vi "SDT_WriteFileDecayFCSMCS.vi"(5 "ActiveModule":string[](array[string]), 7 "FCSFileData":T1, 8 "ErrorIn":errorcluster, 9 "SPCdata":T14={"base_adr"=0, "init"=0, "cfd_limit_low"=0.0, "cfd_limit_high"=0.0, "cfd_zc_level"=0.0, "cfd_holdoff"=0.0, "sync_zc_level"=0.0, "sync_holdoff"=0.0, "sync_threshold"=0.0, "tac_range"=0.0, "sync_freq_div"=0, "tac_gain"=0, "tac_offset"=0.0, "tac_limit_low"=0.0, "tac_limit_high"=0.0, "adc_resolution"=12, "ext_latch_delay"=0, "collect_time"=0.0, "display_time"=0.0, "repeat_time"=0.0, "stop_on_time"=0, "stop_on_ovfl"=0, "dither_range"=0, "count_incr"=0, "mem_bank"=0, "dead_time_comp"=0, "scan_control"=0, "routing_mode"=0, "tac_enable_hold"=0.0, "pci_card_no"=0, "mode"=0, "scan_size_x"=0, "scan_size_y"=0, "scan_rout_x"=0, "scan_rout_y"=0, "scan_flyback"=0, "scan_borders"=0, "scan_polarity"=0, "pixel_clock"=0, "line_compression"=0, "trigger"=0, "pixel_time"=0.0, "ext_pixclk_div"=0, "rate_count_time"=0.0, "macro_time_clk"=0, "add_select"=0, "test_eep"=0, "adc_zoom"=0, "img_size_x"=0, "img_size_y"=0, "img_rout_x"=0, "img_rout_y"=0, "xy_gain"=0, "master_clock"=0, "adc_sample_delay"=0, "detector_type"=0, "chan_enable"=0, "chan_slope"=0, "chan_spec_no"=0, "tdc_control"=0, "tdc_offset1"=0.0, "tdc_offset2"=0.0, "tdc_offset3"=0.0, "tdc_offset4"=0.0, "tdc_offset5"=0.0, "tdc_offset6"=0.0, "cfd_th5_tdc"=0.0, "cfd_th6_tdc"=0.0, "cfd_zc5_tdc"=0.0, "cfd_zc6_tdc"=0.0, "future_reserve1"=0, "future_reserve2"=0, "future_reserve3"=0, "future_reserve4"=0}, 10 "FileType":T2=2 items=["non-Fifo"=1, "Fifo"=2, "FifoImage"=3], 11 "SDT-FilePath":path=path "\\\\lab13\\C/Users/jannis/Desktop/ZeissFifo.sdt") -> (0 "ErrorOut":errorcluster)   [LabVIEW 2017]
doc: "This VI writes a SDT-file to disc. The SetUp and the MeasureInfo blocks are created and appended with the data blocks. \nThis VI is limited to writing a DecayMatrix from a FIFO-Image recording and optional an IntensityImage to file. For single mode recordings use the spcmdll VI \\Public\\Configure\\Memory Transfer\\SPC_save_data_to_sdtfile.vi.\nFor a description of the format for the Data input cluster to this VI see the usage in \\Example\\ImagingEventStream-SimpleFifoImage.vi. Leave either of the cluster input arrays empty to not save them to disc.\nFor a description of the *.sdt file format see: SPC_data_file_structure.h\n\ninfo@becker-hickl.com"
uses:
  SPC_Wrappers/SPC_Controls/bhfile_header.ctl
  SPC_Wrappers/SPC_Controls/SPCdata.ctl
  SPC_Wrappers/SPC_Controls/MeasureInfo.ctl
  SPC_Wrappers/SPC_Controls/MeasureInfo_PartB.ctl
  SPC_Wrappers/SPC_Controls/MeasStopInfo.ctl
  SPC_Wrappers/SPC_Controls/MeasFCSInfo.ctl
  SPC_Wrappers/SPC_Controls/MeasureInfo_PartE.ctl
  SPC_Wrappers/SPC_Controls/MeasHISTInfo.ctl
  SPC_Wrappers/SPC_Controls/HISTInfoExt.ctl
  SPC_Wrappers/SPC_Controls/MeasureInfo_PartI.ctl
  SPC_Wrappers/SPC_Controls/MeasureInfo_PartK.ctl
  SPC_Wrappers/SPC_Controls/MeasureInfo_PartM.ctl
  SPC_Wrappers/SPC_Controls/BHFileBlockHeader.ctl
  SPC_Wrappers/SPC_Controls/FileType.ctl
  SDT_CreateModTypeString.vi
  SDT_MeasureBlockToString.vi
panel:
  out "Info Block":string
  out "BHFileBlockHeaders":T3[](array[typedef])
  out "MeasureInfos":T4 {"MeasStopInfo"."flags" format="x%x"}
  out "ArrayLengths":i32[](array[numeric])
  out "bhfile_header":T15 {"chksum" format="x%x"; "header_valid" format="x%x"}
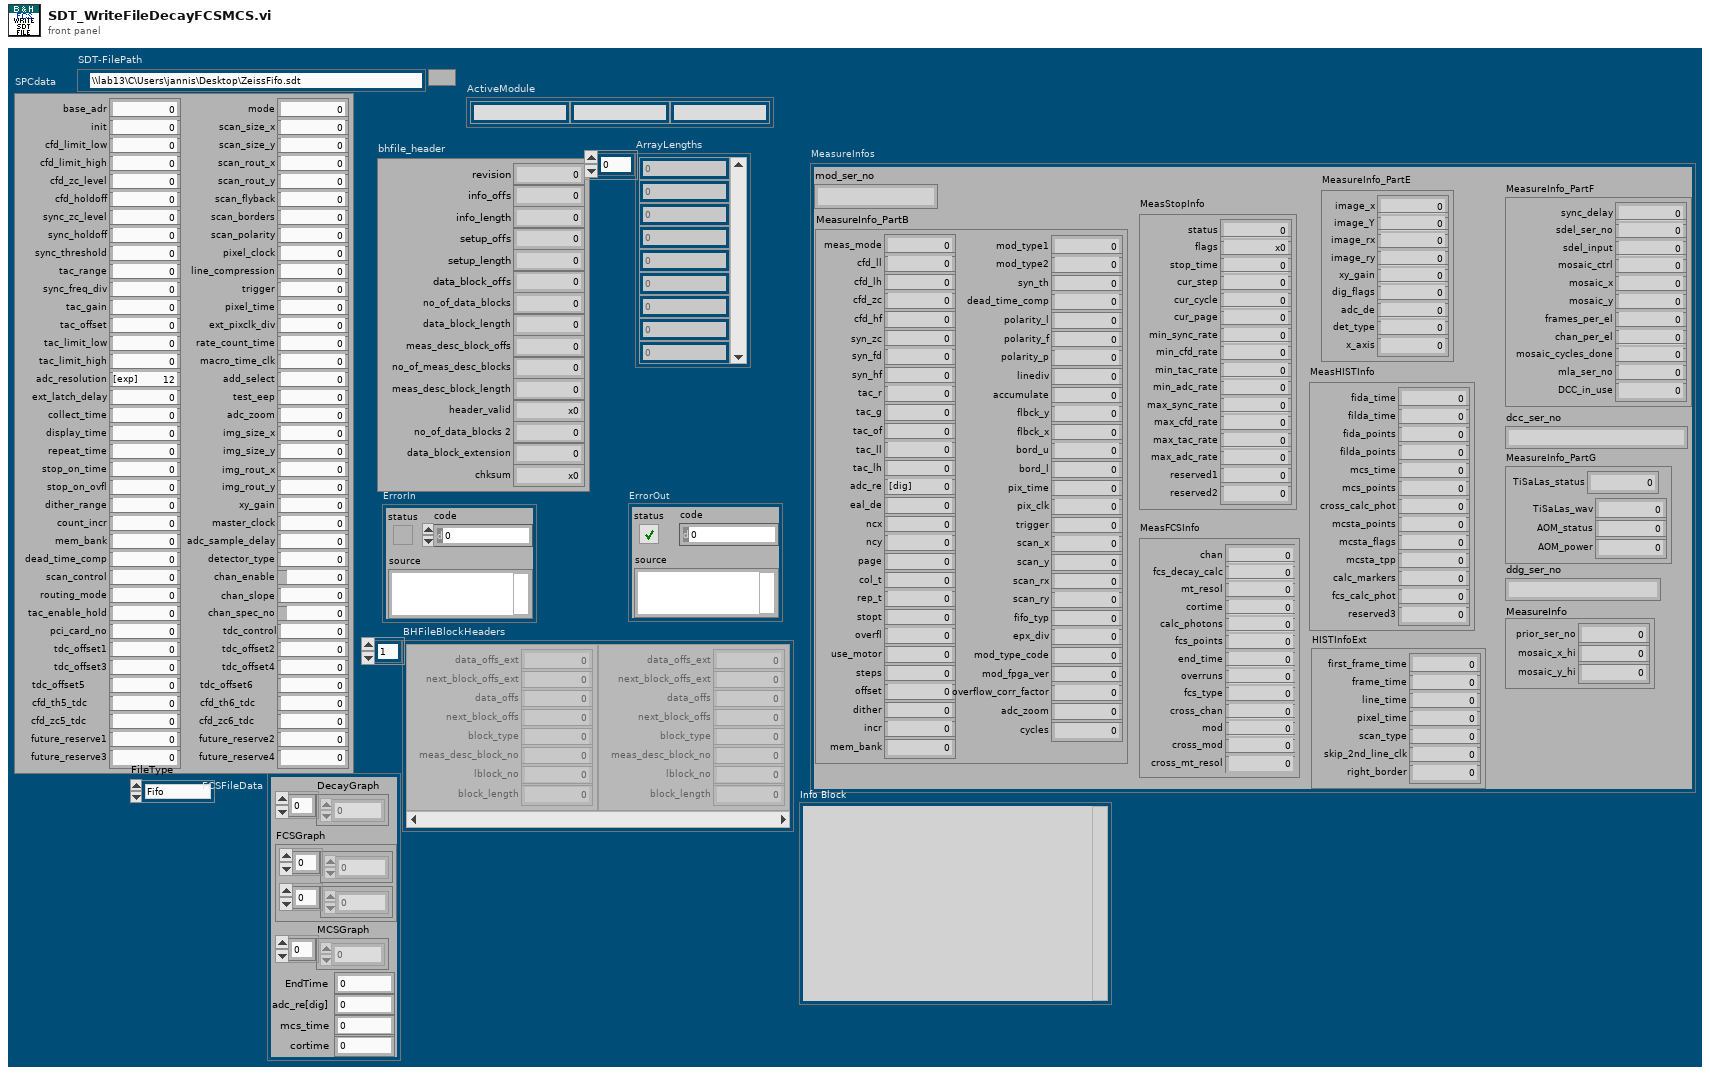
[diagram p1: front panel]
types:
  T1 = cluster{"DecayGraph":i32[], "FCSGraph":cluster{dbl[], dbl[]}, "MCSGraph":u32[], "EndTime":sgl, "adc_re[dig]":i16, "mcs_time":sgl, "cortime":sgl}
  T2 = typedef "FileType.ctl" = u16
  T3 = typedef "BHFileBlockHeader.ctl" = cluster{"data_offs_ext":u8, "next_block_offs_ext":u8, "data_offs":u32, "next_block_offs":u32, "block_type":u16, "meas_desc_block_no":i16, "lblock_no":u32, "block_length":u32}
  T4 = typedef "MeasureInfo.ctl" = cluster{"mod_ser_no":string, "MeasureInfo_PartB":T5, "MeasStopInfo":T6, "MeasFCSInfo":T7, "MeasureInfo_PartE":T8, "MeasHISTInfo":T9, "HISTInfoExt":T10, "MeasureInfo_PartF":T11, "dcc_ser_no":string, "MeasureInfo_PartG":T12, "ddg_ser_no":string, "MeasureInfo":T13}
  T5 = typedef "MeasureInfo_PartB.ctl" = cluster{"meas_mode":i16, "cfd_ll":sgl, "cfd_lh":sgl, "cfd_zc":sgl, "cfd_hf":sgl, "syn_zc":sgl, "syn_fd":i16, "syn_hf":sgl, "tac_r":sgl, "tac_g":i16, "tac_of":sgl, "tac_ll":sgl, "tac_lh":sgl, "adc_re":i16, "eal_de":i16, "ncx":i16, "ncy":i16, "page":u16, "col_t":sgl, "rep_t":sgl, "stopt":i16, "overfl":i8, "use_motor":i16, "steps":u16, "offset":sgl, "dither":i16, "incr":i16, "mem_bank":i16, "mod_type1":u64, "mod_type2":u64, "syn_th":sgl, "dead_time_comp":i16, "polarity_l":i16, "polarity_f":i16, "polarity_p":i16, "linediv":i16, "accumulate":i16, "flbck_y":i32, "flbck_x":i32, "bord_u":i32, "bord_l":i32, "pix_time":sgl, "pix_clk":i16, "trigger":i16, "scan_x":i32, "scan_y":i32, "scan_rx":i32, "scan_ry":i32, "fifo_typ":i16, "epx_div":i32, "mod_type_code":u16, "mod_fpga_ver":u16, "overflow_corr_factor":sgl, "adc_zoom":i32, "cycles":i32}
  T6 = typedef "MeasStopInfo.ctl" = cluster{"status":u16, "flags":u16, "stop_time":sgl, "cur_step":i32, "cur_cycle":i32, "cur_page":i32, "min_sync_rate":sgl, "min_cfd_rate":sgl, "min_tac_rate":sgl, "min_adc_rate":sgl, "max_sync_rate":sgl, "max_cfd_rate":sgl, "max_tac_rate":sgl, "max_adc_rate":sgl, "reserved1":i32, "reserved2":sgl}
  T7 = typedef "MeasFCSInfo.ctl" = cluster{"chan":u16, "fcs_decay_calc":u16, "mt_resol":u32, "cortime":sgl, "calc_photons":u32, "fcs_points":i32, "end_time":sgl, "overruns":u16, "fcs_type":u16, "cross_chan":u16, "mod":u16, "cross_mod":u16, "cross_mt_resol":u32}
  T8 = typedef "MeasureInfo_PartE.ctl" = cluster{"image_x":i32, "image_Y":i32, "image_rx":i32, "image_ry":i32, "xy_gain":i16, "dig_flags":i16, "adc_de":i16, "det_type":i16, "x_axis":i16}
  T9 = typedef "MeasHISTInfo.ctl" = cluster{"fida_time":sgl, "filda_time":sgl, "fida_points":i32, "filda_points":i32, "mcs_time":sgl, "mcs_points":i32, "cross_calc_phot":u32, "mcsta_points":u16, "mcsta_flags":u16, "mcsta_tpp":u32, "calc_markers":u32, "fcs_calc_phot":u32, "reserved3":u32}
  T10 = typedef "HISTInfoExt.ctl" = cluster{"first_frame_time":sgl, "frame_time":sgl, "line_time":sgl, "pixel_time":sgl, "scan_type":i16, "skip_2nd_line_clk":i16, "right_border":u32}
  T11 = typedef "MeasureInfo_PartI.ctl" = cluster{"sync_delay":sgl, "sdel_ser_no":u16, "sdel_input":i8, "mosaic_ctrl":i8, "mosaic_x":u8, "mosaic_y":u8, "frames_per_el":i16, "chan_per_el":i16, "mosaic_cycles_done":i32, "mla_ser_no":u16, "DCC_in_use":u8}
  T12 = typedef "MeasureInfo_PartK.ctl" = cluster{"TiSaLas_status":u16, "TiSaLas_wav":u16, "AOM_status":u8, "AOM_power":u8}
  T13 = typedef "MeasureInfo_PartM.ctl" = cluster{"prior_ser_no":i32, "mosaic_x_hi":u8, "mosaic_y_hi":u8}
  T14 = typedef "SPCdata.ctl" = cluster{"base_adr":u16, "init":i16, "cfd_limit_low":sgl, "cfd_limit_high":sgl, "cfd_zc_level":sgl, "cfd_holdoff":sgl, "sync_zc_level":sgl, "sync_holdoff":sgl, "sync_threshold":sgl, "tac_range":sgl, "sync_freq_div":i16, "tac_gain":i16, "tac_offset":sgl, "tac_limit_low":sgl, "tac_limit_high":sgl, "adc_resolution":i16, "ext_latch_delay":i16, "collect_time":sgl, "display_time":sgl, "repeat_time":sgl, "stop_on_time":i16, "stop_on_ovfl":i16, "dither_range":i16, "count_incr":i16, "mem_bank":i16, "dead_time_comp":i16, "scan_control":u16, "routing_mode":u16, "tac_enable_hold":sgl, "pci_card_no":i16, "mode":u16, "scan_size_x":u32, "scan_size_y":u32, "scan_rout_x":u32, "scan_rout_y":u32, "scan_flyback":u32, "scan_borders":u32, "scan_polarity":u16, "pixel_clock":u16, "line_compression":u16, "trigger":u16, "pixel_time":sgl, "ext_pixclk_div":u32, "rate_count_time":sgl, "macro_time_clk":i16, "add_select":i16, "test_eep":i16, "adc_zoom":i16, "img_size_x":u32, "img_size_y":u32, "img_rout_x":u32, "img_rout_y":u32, "xy_gain":i16, "master_clock":i16, "adc_sample_delay":i16, "detector_type":i16, "chan_enable":u32, "chan_slope":u32, "chan_spec_no":u32, "tdc_control":u32, "tdc_offset1":sgl, "tdc_offset2":sgl, "tdc_offset3":sgl, "tdc_offset4":sgl, "tdc_offset5":sgl, "tdc_offset6":sgl, "cfd_th5_tdc":sgl, "cfd_th6_tdc":sgl, "cfd_zc5_tdc":sgl, "cfd_zc6_tdc":sgl, "future_reserve1":u64, "future_reserve2":u64, "future_reserve3":u64, "future_reserve4":u64}
  T15 = typedef "bhfile_header.ctl" = cluster{"revision":i16, "info_offs":i32, "info_length":i16, "setup_offs":i32, "setup_length":u16, "data_block_offs":i32, "no_of_data_blocks":i16, "data_block_length":u32, "meas_desc_block_offs":i32, "no_of_meas_desc_blocks":i16, "meas_desc_block_length":i16, "header_valid":u16, "no_of_data_blocks 2":u32, "data_block_extension":u16, "chksum":u16}
  T16 = enum16{"open", "replace", "create", "open or create", "replace or create", "replace or create with confirmation"}
  T17 = enum16{"big-endian, network order", "native, host order", "little-endian"}
  T18 = typedef "BHModuleType.ctl" = i16
  T19 = typedef "ModuleType.ctl" = i16
  T20 = cluster{"Decay":i32, i32[], "EndTime":sgl, "adc_re[dig]":i16, "mcs_time":sgl, "cortime":sgl}
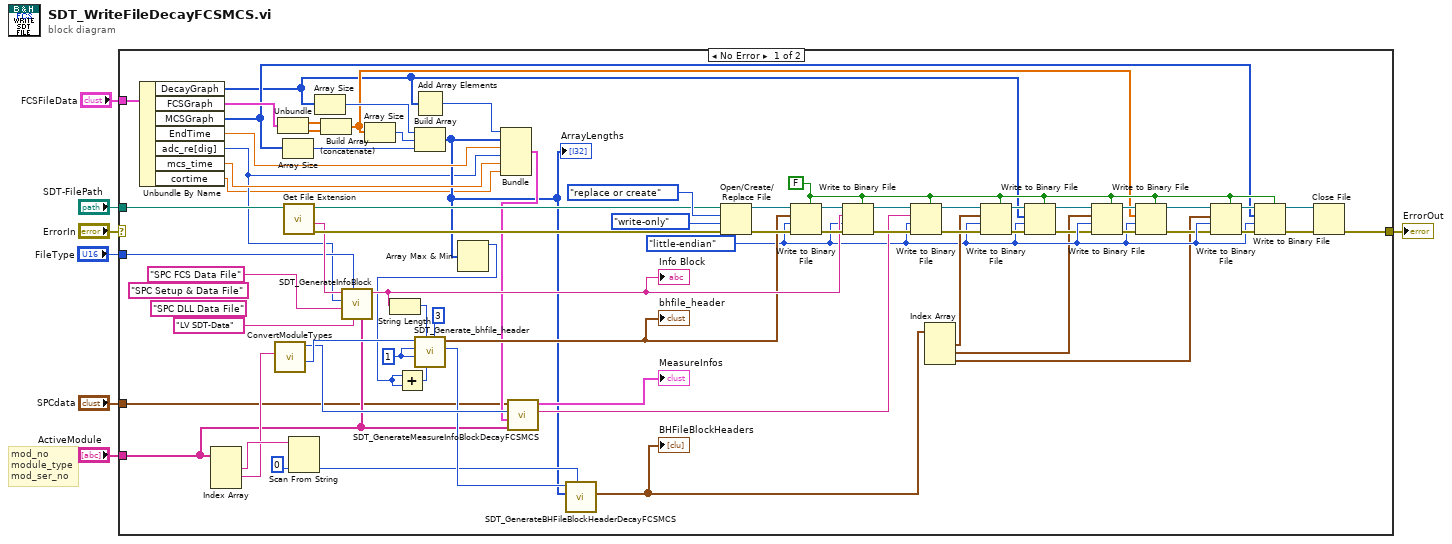
[diagram p0: block diagram]
diagram:
  # "mod_no\nmodule_type\nmod_ser_no"
  n1 = case shown="No Error" "ErrorIn" {
    selector: "ErrorIn" -> [_ w79]
    tunnel: [w8 w79] -> w6
    tunnel: "SPCdata" -> [w9 _]
    tunnel: "ActiveModule" -> [w10 _]
    tunnel: "SDT-FilePath" -> [w54 _]
    tunnel: "FileType" -> [w51 _]
    tunnel: "FCSFileData" -> [w49 _]
    frame No Error {
      (unwired) "SPC Setup & Data File" ("FileID")
      w46 = u32 1 ("ImageSize")
      (unwired) "SPC DLL Data File" ("FileID")
      w37 = FALSE ("prepend array or string size? (T)")
      w36 = T17."little-endian" ("byte order (0:big-endian, network order)")
      n2 = Unbundle By Name(w49) -> ("DecayGraph"=w20:i32[], "FCSGraph"=w26:cluster{dbl[], dbl[]}, "MCSGraph"=w24:u32[], "EndTime"=w17:sgl, "adc_re[dig]"=w13:i16, "mcs_time"=w16:sgl, "cortime"=w11:sgl)
      n3 = Index Array(array=w10) -> (element #1=w69:string, element #2=w67:string)  [unwired: 3 in, 1 out]
      n4 = call "ConvertModuleTypes.vi"("ModuleTypeStringIn"=w67) -> ("BHModuleType"=w60:T18, "Module TypeOut"=w59:T19)  [unwired: 8 in, 1 out]
      n5 = Unbundle(w26) -> (w28:dbl[], w27:dbl[])
      n6 = Array Size(array=w24) -> (size(s)=w23:i32)
      n7 = call <vilib>:"Get File Extension.vi"("file"=w54) -> ("error out"=w73:errorcluster, "filename without extension"=w64:string, "dup file"=w50:path)  [unwired: 6 in, 2 out]
      n8 = Scan From String(input string=w69, default 1=u32 0 ("meas_desc_block_no")) -> (output 1=w55:u32)  [unwired: 3 in, 3 out]
      n9 = Array Size(array=w20) -> (size(s)=w48:i32)
      n10 = Build Array (concatenate)(w28, w27) -> (w25:dbl[])
      n11 = call "SDT_GenerateInfoBlock.vi"("ActiveModule"=w10, "Contents"="LV SDT-Data", "FileType"=w51, "FileID"="SPC FCS Data File", "adc_re[exp]"=w13, "FilenameNoExtension"=w64) -> ("Info Block"=w62:string)  [unwired: 5 in]
      "Info Block" <- w62
      n12 = Array Size(array=w25) -> (size(s)=w21:i32)
      n13 = String Length(string=w62) -> (length=w61:i32)
      n14 = Add Array Elements(numeric array=w20) -> (sum=w19:i32)
      n15 = Build Array(w48, w21, w23) -> (w14:i32[])
      "ArrayLengths" <- w14
      n16 = Array Max & Min(array=w14) -> (max value=w12:i32)  [unwired: 3 out]
      n17 = Add(x=w12, y=w12) -> (x+y=w15:i32)
      n18 = call "SDT_Generate_bhfile_header.vi"("no_of_data_blocks"=u32 3, "adc_re[dig]"=w15, "info_length"=w61, "ImageSize"=w46, "NoOfRoutingChannel"=w46, "BHModuleType"=w60) -> ("data_block_offs"=w56:i32, "bhfile_header"=w57:T15)  [unwired: 4 in]
      "bhfile_header" <- w57
      n19 = Bundle("Decay"=w19, w14, "EndTime"=w17, "adc_re[dig]"=w13, "mcs_time"=w16, "cortime"=w11) -> (w18:T20)  [unwired: 1 in]
      n20 = call "SDT_GenerateMeasureInfoBlockDecayFCSMCS.vi"("ActiveModule"=w10, "MeasureInfoData"=w18, "Module Type"=w59, "SPCdata"=w9) -> ("MeasureInfoStrings"=w53:string, "MeasureInfos"=→"MeasureInfos":T4)  [unwired: 6 in]
      n21 = call "SDT_GenerateBHFileBlockHeaderDecayFCSMCS.vi"("ModuleNo"=w55, "ArrayLengths"=w14, "data_block_offs"=w56) -> ("BHFileBlockHeaders"=w42:T3[])  [unwired: 7 in, 1 out]
      "BHFileBlockHeaders" <- w42
      n22 = Open/Create/Replace File(file path (use dialog)=w50, error in=w73, operation (0:open)=T16."replace or create", access (0:read/write)=enum16{"read/write", "read-only", "write-only"}."write-only") -> (refnum out=w76:refnum<file>, error out=w72:errorcluster)  [unwired: 2 in, 1 out]
      n23 = Write to Binary File(file (use dialog)=w76, data=w57, error in=w72, 5:w37, 9:w36) -> (refnum out=w75:refnum<file>, error out=w71:errorcluster)  [unwired: 1 in, 1 out]
      n24 = Write to Binary File(file (use dialog)=w75, data=w62, error in=w71, 5:w37, 9:w36) -> (refnum out=w74:refnum<file>, error out=w70:errorcluster)  [unwired: 1 in, 1 out]
      n25 = Write to Binary File(file (use dialog)=w74, data=w53, error in=w70, 5:w37, 9:w36) -> (refnum out=w66:refnum<file>, error out=w65:errorcluster)  [unwired: 1 in, 1 out]
      n26 = Index Array(array=w42) -> (element #1=w45:T3, element #2=w32:T3, element #3=w22:T3)  [unwired: 3 in]
      n27 = Write to Binary File(file (use dialog)=w66, data=w45, error in=w65, 5:w37, 9:w36) -> (refnum out=w44:refnum<file>, error out=w43:errorcluster)  [unwired: 1 in, 1 out]
      n28 = Write to Binary File(file (use dialog)=w44, data=w20, error in=w43, 5:w37, 9:w36) -> (refnum out=w31:refnum<file>, error out=w35:errorcluster)  [unwired: 1 in, 1 out]
      n29 = Write to Binary File(file (use dialog)=w31, data=w32, error in=w35, 5:w37, 9:w36) -> (refnum out=w40:refnum<file>, error out=w41:errorcluster)  [unwired: 1 in, 1 out]
      n30 = Write to Binary File(file (use dialog)=w40, data=w25, error in=w41, 5:w37, 9:w36) -> (refnum out=w30:refnum<file>, error out=w34:errorcluster)  [unwired: 1 in, 1 out]
      n31 = Write to Binary File(file (use dialog)=w30, data=w22, error in=w34, 5:w37, 9:w36) -> (refnum out=w39:refnum<file>, error out=w38:errorcluster)  [unwired: 1 in, 1 out]
      n32 = Write to Binary File(file (use dialog)=w39, data=w24, error in=w38, 5:w37, 9:w36) -> (refnum out=w29:refnum<file>, error out=w33:errorcluster)  [unwired: 1 in, 1 out]
      n33 = Close File(refnum=w29, error in=w33) -> (error out=w8:errorcluster)  [unwired: 1 out]
    }
    frame Error {
    }
  }
  "ErrorOut" <- w6
